vi "Kill Task.vi"   [LabVIEW 2014]
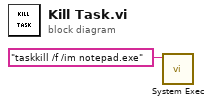
[diagram p0: block diagram]
diagram:
  n1 = call <vilib>:"System Exec.vi"("command line"="taskkill /f /im notepad.exe") -> ()  [unwired: 7 in, 4 out]
